vi "subDFD_Open LabVIEW Project.vi"(11 "lvproj Path":path) -> (0 "error out":errorcluster)   [LabVIEW 2023]
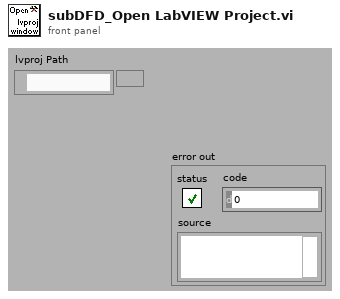
[diagram p1: front panel]
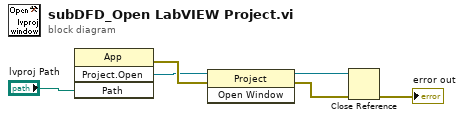
[diagram p0: block diagram]
diagram:
  n1 = invoke class="App" method="Project.Open"("Path"="lvproj Path") -> (error out=w6:errorcluster, "Project:Open"=w3:refnum<vi>)  [unwired: 3 in, 2 out]
  n2 = invoke class="Project" method="Open Window"(reference=w3, error in=w6) -> (reference out=w4:refnum<vi>, error out=w5:errorcluster)  [unwired: 1 in, 1 out]
  n3 = Close Reference(reference=w4, error in (no error)=w5) -> (error out=→"error out":errorcluster)
